vi "Configure Voltage Limit.vi"(6 "Settle (1mS)":u32=1, 8 "error in (no error)":errorcluster, 10 "Voltage Limit (0V)":dbl format="%.4f", 11 "VISA resource name":refnum<visa-resource-name>) -> (0 "error out":errorcluster, 3 "VISA resource name out":refnum<visa-resource-name>)   [LabVIEW 2018, in "TDK-Lambda Z.lvlib"]
doc: "Sets the voltage limit. The power supply output will go to this limit if the load causes Constant-Voltage operation.\n\nNote: This VI will wait for \"Settle\" milliseconds after setting the limit to allow the output to reach the new setting. If unwired, there will be no delay"
uses:
  TDK-Lambda Z.lvlib
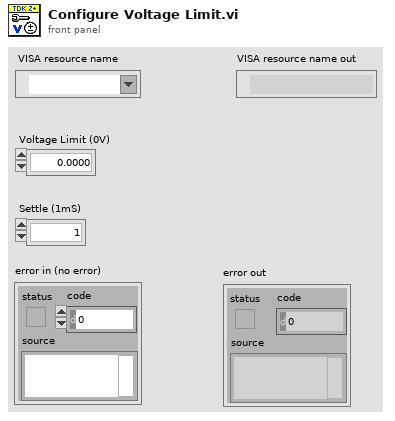
[diagram p1: front panel]
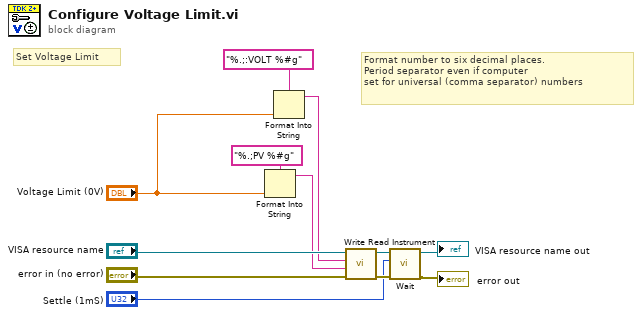
[diagram p0: block diagram]
diagram:
  # "Format number to six decimal places.\nPeriod separator even if computer \nset for universal (comma separator) numbers"
  # "Set Voltage Limit"
  n1 = Format Into String(format string="%.;PV %#g", "Voltage Limit (0V)") -> (resulting string=w7:string)  [unwired: 2 in, 1 out]
  n2 = Format Into String(format string="%.;:VOLT %#g", "Voltage Limit (0V)") -> (resulting string=w10:string)  [unwired: 2 in, 1 out]
  n3 = call "Write Read Instrument.vi"("error in (no error)"="error in (no error)", "GEN  Write Command/Query"=w7, "SCPI  Write Command/Query"=w10, "VISA resource name"="VISA resource name") -> ("error out"=w4:errorcluster, "VISA resource name out"=w5:refnum<visa-resource-name>)  [unwired: 5 in, 1 out]
  n4 = call "Wait.vi"("error in (no error)"=w4, "Wait (1mS)"="Settle (1mS)", "VISA resource name"=w5) -> ("error out"=→"error out":errorcluster, "VISA resource name out"=→"VISA resource name out":refnum<visa-resource-name>)  [unwired: 7 in]
